vi "Check Error.vi"(8 "error in (no error)":errorcluster, 11 "Stop from Queue":bool) -> (0 "error out":errorcluster, 3 "Stop?":bool)   [LabVIEW 2016, in "System.lvlib"]
uses:
  System.lvlib
  Controls/Control_Error Data.ctl
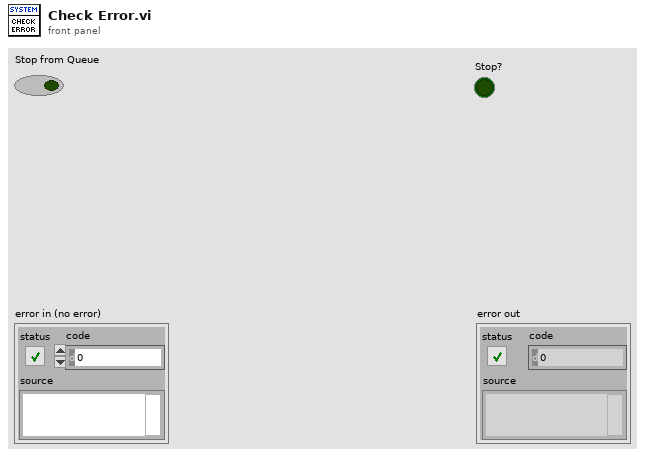
[diagram p1: front panel]
types:
  T1 = typedef "System.lvlib/Control_Error Data.ctl" = cluster{"Time":timestamp, "Error":errorcluster}
  T2 = typedef "System.lvlib/Control_User Event.ctl" = cluster{"Stop":refnum<user-event>, "Error":refnum<user-event>}
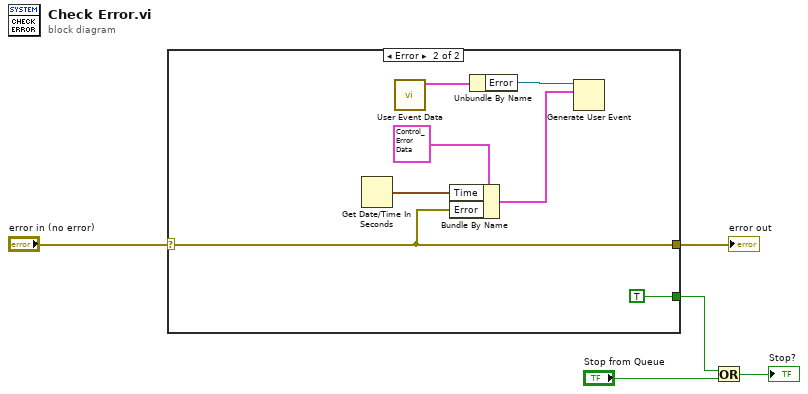
[diagram p0: block diagram]
diagram:
  n1 = case shown="Error" "error in (no error)" {
    selector: "error in (no error)" -> [w6 w8]
    tunnel: [w6 w8] -> w4
    tunnel: [_ TRUE] -> w2
    frame No Error {
    }
    frame Error {
      n2 = Get Date/Time In Seconds() -> (seconds since 1Jan1904=w9:timestamp)
      n3 = call "User Event Data.vi"() -> ("User Event Data"=w12:T2)  [unwired: 10 in, 1 out]
      n4 = Bundle By Name(cluster=T1 {"Time"=timestamp(0 s since 1904-01-01), "Error"={"status"=FALSE, "code"=0, "source"=""}} ("Error Data"), "Time"=w9, "Error"=w8) -> (w7:T1)
      n5 = Unbundle By Name(w12) -> ("Error"=w11:refnum<user-event>)
      n6 = Generate User Event(user event=w11, event data cluster=w7) -> ()  [unwired: 2 in, 2 out]
    }
  }
  "error out" <- w4
  n7 = Or(x=w2, y="Stop from Queue") -> (x .or. y?=→"Stop?":bool)
